vi "Create Subset String Buffer.vi"(8 "error in (no error)":errorcluster, 9 "offset":u64 format="%d bytes", 10 "size":u64 format="%d bytes", 11 "Framework in":refnum<class "Framework.lvclass">) -> (0 "error out":errorcluster, 1 "offset + size":u64 format="%d bytes", 2 "subset String Buffer":refnum<class "Buffer.lvclass">, 3 "Framework out":refnum<class "Framework.lvclass">)   [LabVIEW 2017, in "DSF Core.lvlib" / "Framework.lvclass"]
uses:
  Framework.lvclass
  <vilib>/NI/Memory Manager/Classes/Pointer/Memory.Pointer.lvclass
  Buffer/Buffer.lvclass
  C:/Program Files (x86)/National Instruments/LabVIEW 2017/vi.lib/NI/Memory Manager/Classes/Pointer/Memory.Pointer.lvclass
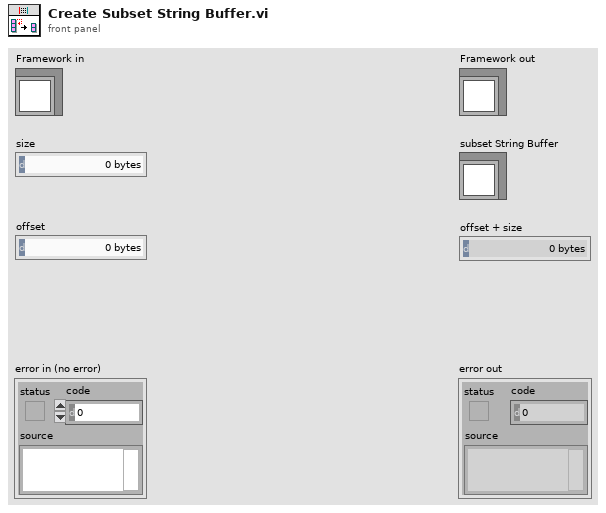
[diagram p1: front panel]
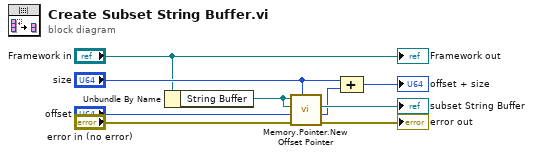
[diagram p0: block diagram]
diagram:
  n1 = Unbundle By Name("Framework in") -> ("String Buffer"=w9:refnum<class "Buffer.lvclass">)
  n2 = call <vilib>:"Memory.Pointer.New Offset Pointer.vi"("length (-1: rest)"="size", "error in (no error)"="error in (no error)", "offset (0)"="offset", "offset Pointer type"=w9, "base Pointer in"=w9) -> ("error out"=→"error out":errorcluster, "offset out"=w3:u64, "offset Pointer"=→"subset String Buffer":refnum<class "Buffer.lvclass">)  [unwired: 3 in, 1 out]
  n3 = Compound Arithmetic op=ADD("size", w3) -> (→"offset + size":u64)
  "Framework out" <- "Framework in"
